vi "prueba1_240.vi"() -> ()   [LabVIEW 2011]
panel:
  out "Tanque":i32(slide) scale=1.0..1000.0
  out "601-1000 LLENO":bool
  out "301-600 MEDIO":bool
  out "1-300 VACIO":bool
  # "EL PROGRAMA DEBERA DE LLENAR EL TANQUE \nLA BOMBA GENERA DE 1-50 GALONES. LOS CUALES SE SUMAN \nY ESTA SUMA SE REPRESENTA POR EL TANQUE.\nDEBERA DE IR ENCENDIENDO LOS LED DE ACUERDO \nAL VOLUMEN DE AGUA DEL TANQUE \nCUANDO ESTE SE LLENE SE DETIENE EL PROGRAMA \nNOTA LLENADO SE ENTIENDE CUANDO LA SUMA ES IGUAL O MAYOR"
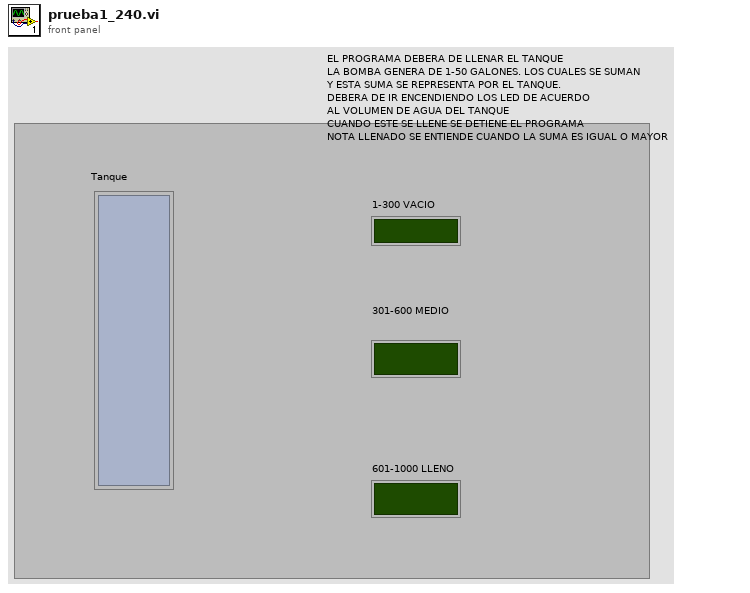
[diagram p1: front panel]
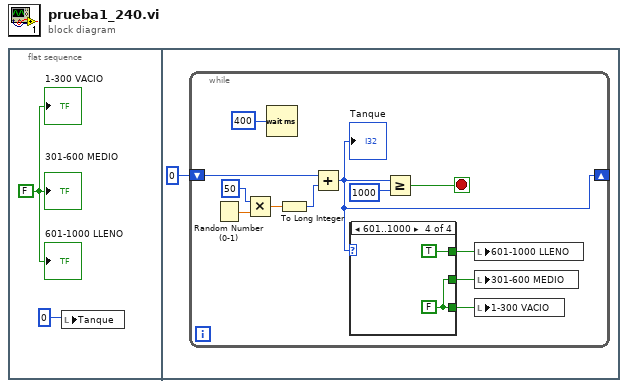
[diagram p0: block diagram]
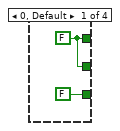
[diagram p2: hidden frame]
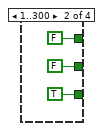
[diagram p3: hidden frame]
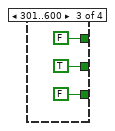
[diagram p4: hidden frame]
diagram:
  n1 = flat-sequence {
    frame #0 {
      w2 = FALSE
      n2 = local write "Tanque"(0) -> ()
      "1-300 VACIO" <- w2
      "301-600 MEDIO" <- w2
      "601-1000 LLENO" <- w2
    }
    frame #1 {
      n3 = while {
        shift-right: [w4] -> _
        shift-left: 0 -> [w12]
        stop <- w7 stop-if-true
        n4 = Random Number (0-1)() -> (number: 0 to 1=w15:dbl)
        n5 = Multiply(x=50, y=w15) -> (x*y=w13:dbl)
        n6 = Wait (ms)(milliseconds to wait=400) -> ()  [unwired: 1 out]
        n7 = To Long Integer(number=w13) -> (32bit integer=w6:i32)
        n8 = Add(x=w12, y=w6) -> (x+y=w4:i32)
        "Tanque" <- w4
        n9 = case shown="601..1000" w4 {
          tunnel: [FALSE TRUE FALSE w25] -> w8
          tunnel: [w16 FALSE TRUE w25] -> w9
          tunnel: [w16 FALSE FALSE TRUE] -> w10
          frame 0, Default {
            w16 = FALSE
          }
          frame 1..300 {
          }
          frame 301..600 {
          }
          frame 601..1000 {
            w25 = FALSE
          }
        }
        n10 = Greater Or Equal?(x=w4, y=1000) -> (x >= y?=w7:bool)
        n11 = local write "601-1000 LLENO"(w10) -> ()
        n12 = local write "301-600 MEDIO"(w9) -> ()
        n13 = local write "1-300 VACIO"(w8) -> ()
      }
    }
  }
